vi "Write Timer.vi"(8 "error in (no error)":errorcluster, 10 "Timer":u32, 11 "SPARC4_GUI in":refnum<class "S4GEI.lvclass">) -> (0 "error out":errorcluster, 3 "SPARC4_GUI out":refnum<class "S4GEI.lvclass">)   [LabVIEW 2018, in "S4GEI.lvclass"]
uses:
  S4GEI.lvclass
  S4GEI.lvclass/S4GEI.ctl
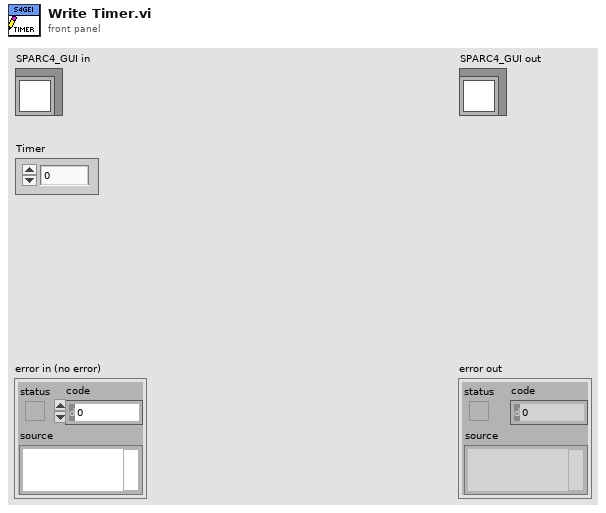
[diagram p1: front panel]
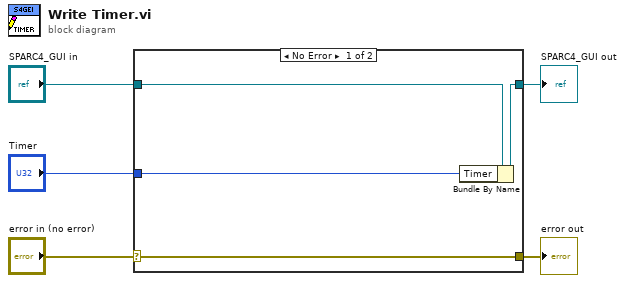
[diagram p0: block diagram]
diagram:
  n1 = case shown="No Error" "error in (no error)" {
    selector: "error in (no error)" -> [w9 w10]
    tunnel: [w9 w10] -> w4
    tunnel: [w7 w11] -> w2
    tunnel: "SPARC4_GUI in" -> [w8 w11]
    tunnel: "Timer" -> [w6 _]
    frame No Error {
      n2 = Bundle By Name(cluster=w8, "Timer"=w6) -> (w7:refnum<class "S4GEI.lvclass">)
    }
    frame Error {
    }
  }
  "error out" <- w4
  "SPARC4_GUI out" <- w2
